vi "prepareStiffnessBaseline.vi"(8 "error in (no error)":errorcluster, 11 "Model in":refnum<class "Model.lvclass">) -> (0 "error out":errorcluster, 3 "Model out":refnum<class "Model.lvclass">)   [LabVIEW 2015]
uses:
  ApplicationElements/StiffnessMonitor/StiffnessMonitor.lvclass
  <userlib>/Common/Devices/ForceSensorCalculator/ForceSensorCalculator/ForceSensorCalculator.lvclass
  <userlib>/Common/Devices/DistanceGauge/DistanceGauge/DistanceGauge.lvclass
  Model.lvclass
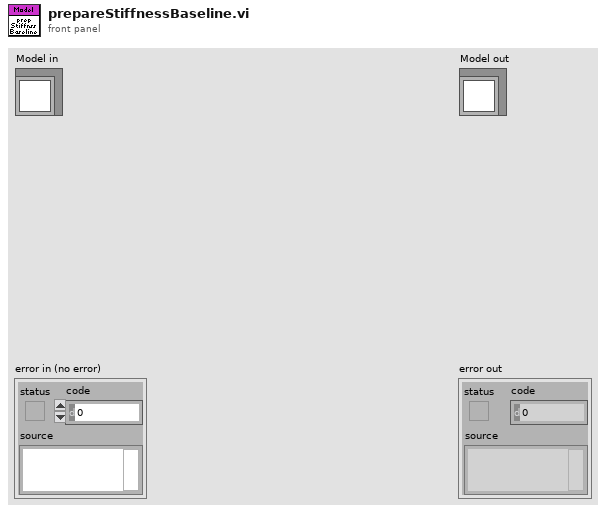
[diagram p1: front panel]
types:
  T1 = typedef "DistanceGauge.lvlib/Distance Data.ctl" = cluster{"Distance Measured":dbl[unit]}
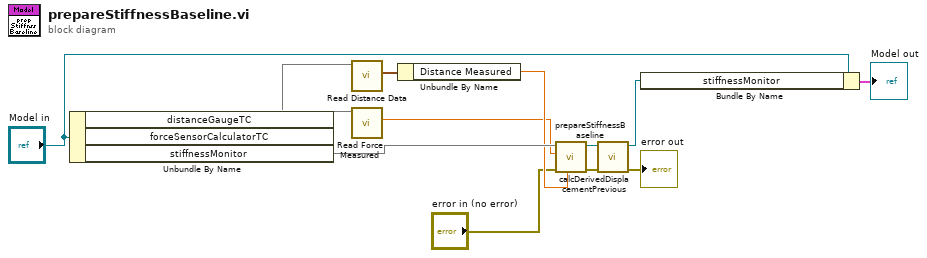
[diagram p0: block diagram]
diagram:
  n1 = Unbundle By Name("Model in") -> ("distanceGaugeTC"=w5, "forceSensorCalculatorTC"=w10, "stiffnessMonitor"=w13)
  n2 = call <userlib>:"Read Distance Data.vi"("DistanceGauge in"=w5) -> ("Distance Data"=w4:T1)  [unwired: 9 in, 1 out]
  n3 = call <userlib>:"Read Force Measured.vi"("ForceSensor in"=w10) -> ("Force Demand"=w9:dbl[unit])  [unwired: 9 in, 1 out]
  n4 = Unbundle By Name(w4) -> ("Distance Measured"=w11:dbl[unit])
  n5 = call "prepareStiffnessBaseline.vi"("Distance to Plate Measured"=w11, "error in (no error)"="error in (no error)", "Force Measured"=w9, "StiffnessMonitor in"=w13) -> ("error out"=w2:errorcluster, "StiffnessMonitor out"=w12:refnum<class "StiffnessMonitor.lvclass">)  [unwired: 6 in]
  n6 = call "calcDerivedDisplacementPrevious.vi"("error in (no error)"=w2, "StiffnessMonitor in"=w12) -> ("error out"=→"error out":errorcluster, "StiffnessMonitor out"=w8:refnum<class "StiffnessMonitor.lvclass">)  [unwired: 8 in]
  n7 = Bundle By Name(cluster="Model in", "stiffnessMonitor"=w8) -> (→"Model out":cluster{})
